vi "ConfigureDlg.vi"(8 "error in (no error)":errorcluster, 11 "RoomAlert in":refnum<class "RoomAlert.lvclass">) -> (0 "error out":errorcluster, 2 "Changed":bool, 3 "RoomAlert out":refnum<class "RoomAlert.lvclass">)   [LabVIEW 2018, in "SensorPlugins.lvlib" / "RoomAlert.lvclass"]
doc: "Configure the instrument using the provided panel and saves the instruments configuration to file, a new file, or cancels the entire operation."
uses:
  RoomAlert.lvclass
  C:/Program Files (x86)/National Instruments/LabVIEW 2018/user.lib/NIST/BaseClasses/BasePlugin_class/BasePlugin.lvclass
  TypeDefinitions/RoomAlertControls.ctl
  TypeDefinitions/MeasurementControls.ctl
  <userlib>/NIST/BaseClasses/BasePlugin_class/BasePlugin.lvclass/BasePlugin.ctl
  <userlib>/NIST/BaseClasses/BasePlugin_class/Accessors/Read PluginIniFilePath.vi
  <userlib>/NIST/BaseClasses/BasePlugin_class/Accessors/Write PluginIniFilePath.vi
  <vilib>/Utility/error.llb/Error Cluster From Error Code.vi
  <vilib>/ErrorRing/Error Ring.xnode
  <vilib>/Utility/config.llb/NI_LVConfig.lvlib
panel:
  in  "Throw Error":bool
  in  "MeasurementCluster":T1={"Measurement RefreshTime (ms)"=1000, "Measurement Name"="Sensor.RoomAlert0", "Timeout(ms)"=5000, "Amber Warning Light Configuration"={"Warning Temperture (Degrees C)"=0.0, "Temperature Delta (Degrees C/Minute)"=0.0, "Time Window (Minutes)"=0.0}}
  in  "RoomAlert Device":T2 {"Measurements To Read Array" items=["Internal Temp F", "Internal Temp C", "Digital Sensor 1 Temp C", "Digital Sensor 1 Temp F", "Digital Sensor 2 Temp C", "Digital Sensor 2 Temp F", "Alarm Message"]}
  in  "btnSaveAs":bool
  in  "btnSave":bool
  in  "btnCancel":bool
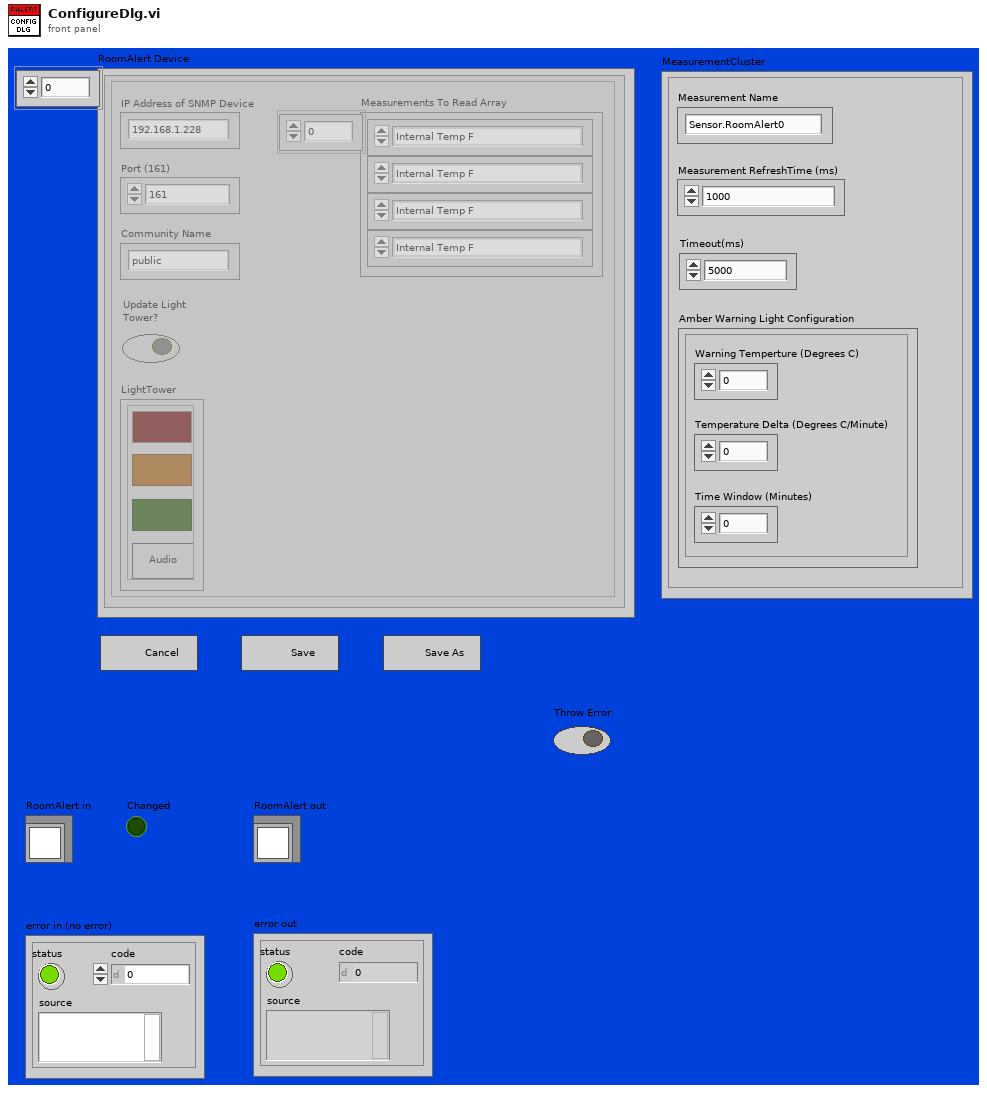
[diagram p1: front panel]
types:
  T1 = typedef "SensorPlugins.lvlib/RoomAlert.lvclass/MeasurementControls.ctl" = cluster{"Measurement RefreshTime (ms)":u32, "Measurement Name":string, "Timeout(ms)":i32, "Amber Warning Light Configuration":cluster{"Warning Temperture (Degrees C)":dbl, "Temperature Delta (Degrees C/Minute)":dbl, "Time Window (Minutes)":dbl}}
  T2 = typedef "SensorPlugins.lvlib/RoomAlert.lvclass/RoomAlertControls.ctl" = cluster{"Connected?":bool, "IP Address of SNMP Device":string, "Port (161)":u16, "Community Name":string, "Measurements To Read Array":u16[], "Update Light \nTower?":bool, "LightTower":cluster{"Red":bool, "Amber":bool, "Green":bool, "Audio":bool}}[]
  T3 = enum32{"Invalid", "Default", "Floating", "Floating/Auto-Hide", "Modal"}
  T4 = enum32{"Invalid", "Standard", "Closed", "Hidden", "Minimized", "Maximized"}
  T5 = enum8{"Enabled", "Disabled", "Disabled and Grayed Out"}
  T6 = cluster{"Connected?":bool, "IP Address of SNMP Device":string, "Port (161)":u16, "Community Name":string, "Measurements To Read Array":u16[], "Update Light \nTower?":bool, "LightTower":cluster{"Red":bool, "Amber":bool, "Green":bool, "Audio":bool}}
  T7 = typedef "NI_LVConfig.lvlib/Config Data RefNum.ctl" = refnum<k1>
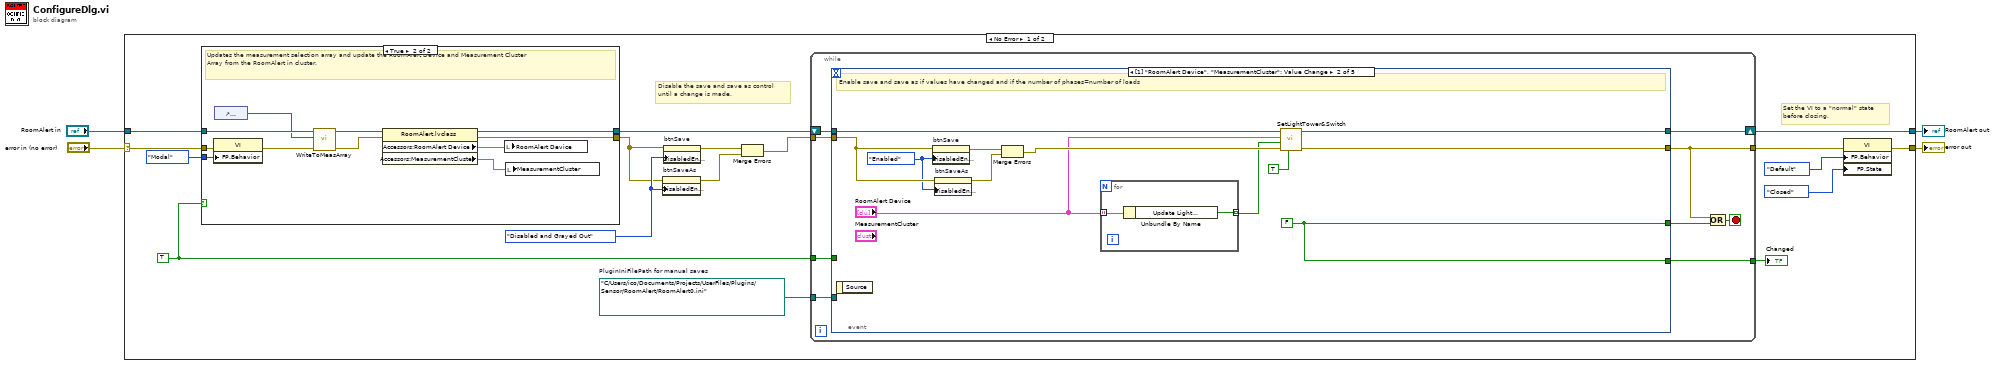
[diagram p0: block diagram]
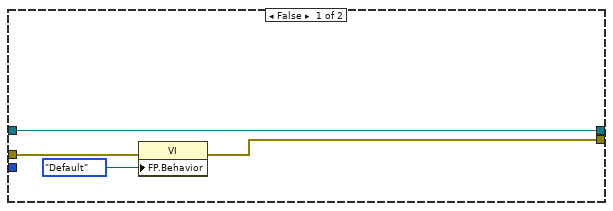
[diagram p2: hidden frame]
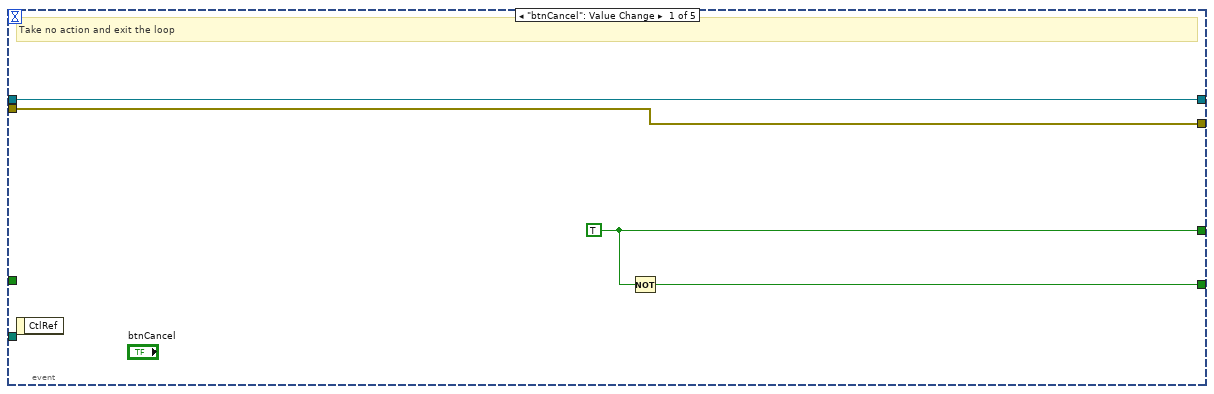
[diagram p3: hidden frame]
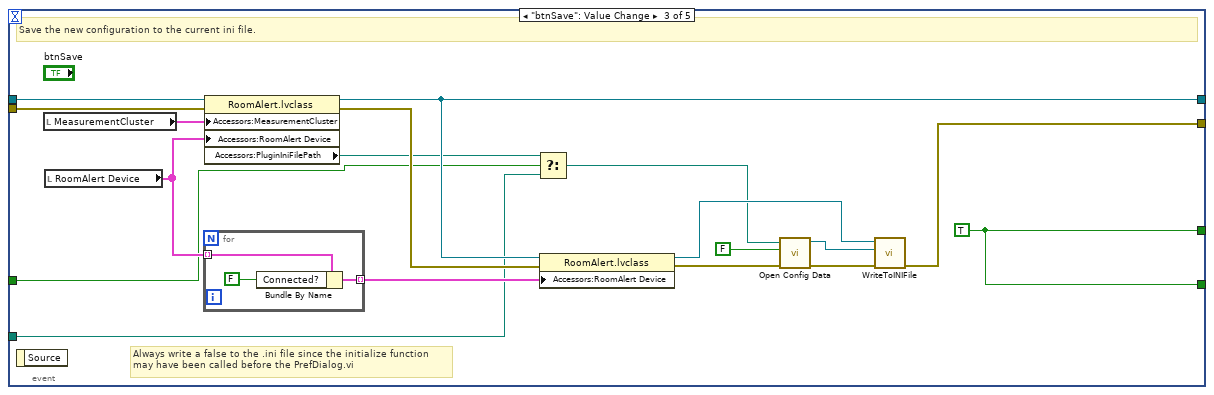
[diagram p4: hidden frame]
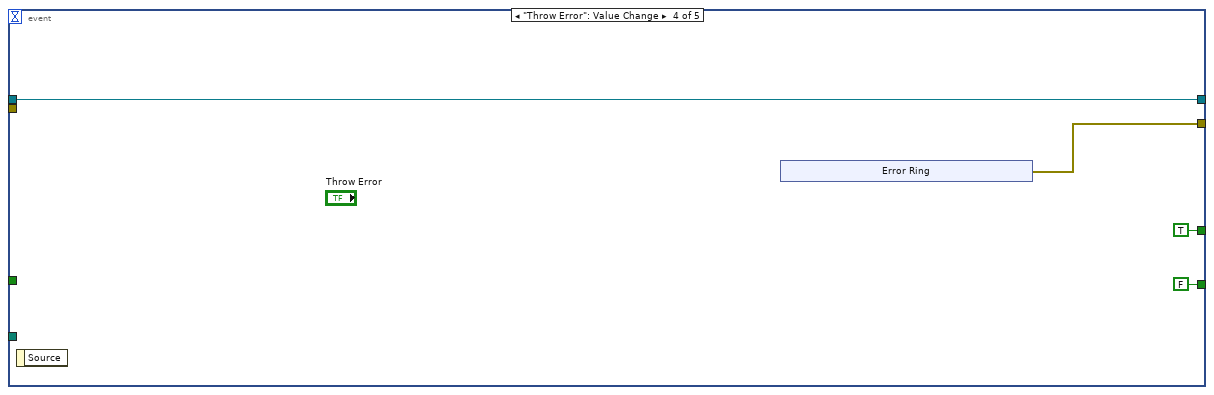
[diagram p5: hidden frame]
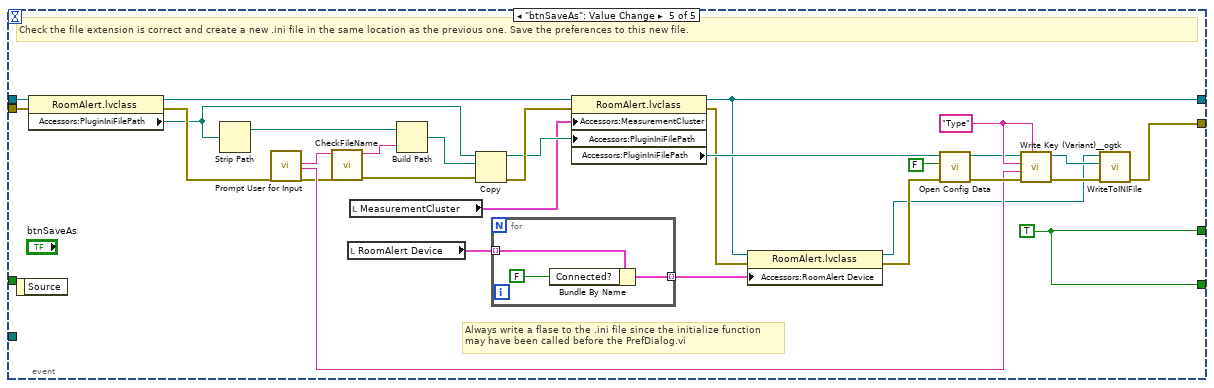
[diagram p6: hidden frame]
diagram:
  n1 = case shown="No Error" "error in (no error)" {
    selector: "error in (no error)" -> [w6 w126]
    tunnel: [w12 w127] -> w2
    tunnel: [w9 w126] -> w1
    tunnel: "RoomAlert in" -> [w7 w127]
    frame No Error {
      w5 = TRUE ("Read from PropertyNode")
      w16 = T5."Disabled and Grayed Out" ("Disabled")
      w13 = path "C:/Users/ico/Documents/Projects/UserFiles/Plugins/Sensor/RoomAlert/RoomAlert0.ini"  # PluginIniFilePath for manual saves
      # "Set the VI to a \"normal\" state\nbefore closing."
      # "Disable the save and save as control\nuntil a change is made."
      n2 = case shown="True" w5 {
        tunnel: T3."Modal" ("Front Panel Window:Behavior") -> [_ w36]
        tunnel: [w25 w35] -> w19
        tunnel: [w23 w34] -> w15
        tunnel: w7 -> [w25 w33]
        tunnel: w6 -> [w24 w32]
        frame False {
          n3 = property class="VI"(error in=w24, "FP.Behavior"=T3."Default" ("Front Panel Window:Behavior")) -> (error out=w23:errorcluster)  [unwired: 1 in, 1 out]
        }
        frame True {
          # "Updates the measurement selection array and update the RoomAlert Device and Measurement Cluster\nArray from the RoomAlert in cluster."
          n4 = property class="VI"(error in=w32, "FP.Behavior"=w36) -> (error out=w31:errorcluster)  [unwired: 1 in, 1 out]
          n5 = control-ref of="RoomAlert Device"() -> (w29:refnum<vi>)
          n6 = call-dynamic "WriteToMeasArray.vi"("error in (no error)"=w31, "RoomAlert Device Reference"=w29, "RoomAlert in"=w33) -> ("error out"=w28:errorcluster, "RoomAlert out"=w30:refnum<class "RoomAlert.lvclass">)  [unwired: 7 in]
          n7 = property class="RoomAlert.lvclass"(reference=w30, error in=w28) -> (reference out=w35:refnum<class "RoomAlert.lvclass">, error out=w34:errorcluster, "Accessors:RoomAlert Device"=w27:T2, "Accessors:MeasurementCluster"=w26:T1)
          n8 = local write "RoomAlert Device"(w27) -> ()
          n9 = local write "MeasurementCluster"(w26) -> ()
        }
      }
      n10 = property on="btnSaveAs" class="Bool"(error in=w15, "DisabledEnum"=w16) -> (error out=w17:errorcluster)  [unwired: 1 in, 1 out]
      n11 = property on="btnSave" class="Bool"(error in=w15, "DisabledEnum"=w16) -> (error out=w18:errorcluster)  [unwired: 1 in, 1 out]
      n12 = Merge Errors(w18, w17) -> (w14:errorcluster)
      n13 = while {
        shift-right: [w44] -> w12
        shift-left: w19 -> [w45]
        tunnel: w14 -> [w43]
        tunnel: [w40] -> w11
        tunnel: [w42] -> w8
        tunnel: w13 -> [w38]
        tunnel: w5 -> [w37]
        stop <- w41 stop-if-true
        n14 = event shown="[1] \"RoomAlert Device\", \"MeasurementCluster\": Value Change" {
          selector: _ -> [_ _ _ _ _]
          dyn-events: _ -> [_ _ _ _ _]
          timeout: _ -> [_ _ _ _ _]
          tunnel: w45 -> [w49 w53 w79 w88 w108]
          tunnel: [w47 w61 w80 TRUE w121] -> w39
          tunnel: [w49 w54 w71 w88 w94] -> w44
          tunnel: w43 -> [w48 w60 w76 _ w107]
          tunnel: [w48 w55 w77 w85 w119] -> w40
          tunnel: [w46 w61 w80 FALSE w121] -> w42
          tunnel: w38 -> [_ _ w68 _ _]
          tunnel: w37 -> [_ _ w64 _ _]
          event "btnCancel": Value Change {
            w47 = TRUE
            # "Take no action and exit the loop"
            n15 = event-data() -> ()  [unwired: 1 in, 1 out]
            n16 = Not(x=w47) -> (.not. x?=w46:bool)
          }
          event Value Change {
            w57 = T5."Enabled" ("Disabled")
            w61 = FALSE
            # "Enable save and save as if values have changed and if the number of phases=number of loads"
            n17 = event-data() -> ()  [unwired: 1 in, 1 out]
            n18 = property on="btnSave" class="Bool"(error in=w60, "DisabledEnum"=w57) -> (error out=w58:errorcluster)  [unwired: 1 in, 1 out]
            n19 = property on="btnSaveAs" class="Bool"(error in=w60, "DisabledEnum"=w57) -> (error out=w59:errorcluster)  [unwired: 1 in, 1 out]
            n20 = Merge Errors(w58, w59) -> (w56:errorcluster)
            n21 = for {
              tunnel: "RoomAlert Device" -> [w63] mode=indexing
              tunnel: [w62] -> w51 mode=indexing
              n22 = Unbundle By Name(w63) -> ("Update Light \nTower?"=w62:bool)
            }
            n23 = call-dynamic "SetLightTower&Switch.vi"("Supress Match Error (F)"=TRUE, "error in (no error)"=w56, "UpdateValue? (F)"=w51, "RoomAlert Device"="RoomAlert Device", "RoomAlert in"=w53) -> ("error out"=w55:errorcluster, "RoomAlert out"=w54:refnum<class "RoomAlert.lvclass">)  [unwired: 5 in]
          }
          event "btnSave": Value Change {
            w80 = TRUE
            # "Always write a false to the .ini file since the initialize function\nmay have been called before the PrefDialog.vi"
            # "Save the new configuration to the current ini file."
            n24 = event-data() -> ()  [unwired: 1 in, 1 out]
            n25 = local read "MeasurementCluster"() -> (w65:T1)
            n26 = local read "RoomAlert Device"() -> (w66:T2)
            n27 = for {
              tunnel: w66 -> [w83] mode=indexing
              tunnel: [w84] -> w74 mode=indexing
              n28 = Bundle By Name(cluster=w83, "Connected?"=FALSE) -> (w84:T6)
            }
            n29 = property class="RoomAlert.lvclass"(reference=w79, error in=w76, "Accessors:MeasurementCluster"=w65, "Accessors:RoomAlert Device"=w66) -> (reference out=w71:refnum<class "RoomAlert.lvclass">, error out=w75:errorcluster, "Accessors:PluginIniFilePath"=w69:path)
            n30 = Select(t=w69, s=w64, f=w68) -> (s? t:f=w67:path)
            n31 = property class="RoomAlert.lvclass"(reference=w71, error in=w75, "Accessors:RoomAlert Device"=w74) -> (reference out=w70:refnum<class "RoomAlert.lvclass">, error out=w72:errorcluster)
            n32 = call <vilib>:"Open Config Data.vi"("error in (no error)"=w72, "create file if necessary (T)"=FALSE, "configuration file path"=w67) -> ("error out"=w73:errorcluster, "refnum"=w78:T7)  [unwired: 6 in, 1 out]
            n33 = call-dynamic "WriteToINIFile.vi"("error in (no error)"=w73, "Refnum in"=w78, "RoomAlert in"=w70) -> ("error out"=w77:errorcluster)  [unwired: 7 in, 1 out]
          }
          event "Throw Error": Value Change {
            n34 = event-data() -> ()  [unwired: 1 in, 1 out]
            n35 = xnode "Error Ring"() -> ("error out"=w85:errorcluster)
          }
          event "btnSaveAs": Value Change {
            w118 = "Type" ("section (optional)")
            w121 = TRUE
            # "Always write a flase to the .ini file since the initialize function\nmay have been called before the PrefDialog.vi"
            # "Check the file extension is correct and create a new .ini file in the same location as the previous one. Save the preferences to this new file."
            n36 = event-data() -> ()  [unwired: 1 in, 1 out]
            n37 = property class="RoomAlert.lvclass"(reference=w108, error in=w107) -> (reference out=w106:refnum<class "RoomAlert.lvclass">, error out=w105:errorcluster, "Accessors:PluginIniFilePath"=w104:path)
            n38 = Strip Path(path=w104) -> (stripped path=w113:path)  [unwired: 1 out]
            n39 = call "Prompt User for Input"("error in (no error)"=w105) -> ("File Name"=w100:string, "PluginType"=w103:string, "error out"=w99:errorcluster)  [unwired: 15 in, 1 out]
            n40 = call "CheckFileName.vi"("Error In"=w99, "File Name in"=w100) -> ("Error Out"=w101:errorcluster, "File Name out"=w102:string)  [unwired: 8 in]
            n41 = local read "RoomAlert Device"() -> (w120:T2)
            n42 = local read "MeasurementCluster"() -> (w98:T1)
            n43 = Build Path(base path=w113, name or relative path=w102) -> (appended path=w112:path)
            n44 = Copy(8:w101, 10:w112, 11:w104) -> (0:w111:errorcluster, 3:w109:path)  [unwired: 2 in, 1 out]
            n45 = for {
              tunnel: w120 -> [w124] mode=indexing
              tunnel: [w125] -> w97 mode=indexing
              n46 = Bundle By Name(cluster=w124, "Connected?"=FALSE) -> (w125:T6)
            }
            n47 = property class="RoomAlert.lvclass"(reference=w106, error in=w111, "Accessors:MeasurementCluster"=w98, "Accessors:PluginIniFilePath"=w109) -> (reference out=w94:refnum<class "RoomAlert.lvclass">, error out=w96:errorcluster, "Accessors:PluginIniFilePath"=w110:path)
            n48 = property class="RoomAlert.lvclass"(reference=w94, error in=w96, "Accessors:RoomAlert Device"=w97) -> (reference out=w93:refnum<class "RoomAlert.lvclass">, error out=w95:errorcluster)
            n49 = call <vilib>:"Open Config Data.vi"("error in (no error)"=w95, "create file if necessary (T)"=FALSE, "configuration file path"=w110) -> ("error out"=w116:errorcluster, "refnum"=w117:T7)  [unwired: 6 in, 1 out]
            n50 = call <userlib>:"Write Key (Variant)__ogtk.vi"("section"=w118, "error in (no error)"=w116, "key-value"=w103, "key (optional)"=w118, "refnum"=w117) -> ("error out"=w115:errorcluster, "refnum out"=w114:T7)  [unwired: 5 in]
            n51 = call-dynamic "WriteToINIFile.vi"("error in (no error)"=w115, "Refnum in"=w114, "RoomAlert in"=w93) -> ("error out"=w119:errorcluster)  [unwired: 7 in, 1 out]
          }
        }
        n52 = Or(x=w40, y=w39) -> (x .or. y?=w41:bool)
      }
      "Changed" <- w8
      n53 = property class="VI"(error in=w11, "FP.Behavior"=T3."Default" ("Front Panel Window:Behavior"), "FP.State"=T4."Closed" ("Front Panel Window:State")) -> (error out=w9:errorcluster)  [unwired: 1 in, 1 out]
    }
    frame Error {
    }
  }
  "error out" <- w1
  "RoomAlert out" <- w2
